vi "main_FP.vi"() -> ()   [LabVIEW 2011]
uses:
  global.vi
  <vilib>/Instr/_visa.llb/VISA Configure Serial Port (Instr).vi
panel:
  in  "EXIT":bool caption="Start_reception"
  out "status_error":bool caption="status_rx"
  out "status_tx":bool
  out "status_rx":bool
  out "status_connected":bool
  in  "Main tab":T1(tab)
  in  "Stop_rx":bool
  out "Receiving":bool
  out "Signal Noise Ratio":string="0"
  out "Packet number":i32
  in  "Start_reception":bool
  in  "reception_list":i32(listbox)
  out "reception Graph":dbl[](graph)
  in  "Stop_tx":bool
  out "Transmitting":bool
  in  "Delay between packets (ms)":u32=2000 max=65535 step=1
  in  "tx_timestamp":bool=TRUE caption="Add timestamp"
  in  "tx_packetnum":bool=TRUE caption="Add packet number"
  in  "Message":string="Aloha"
  out "TX Packet number":i32 caption="Packet number"
  in  "Start_transmission":bool
  in  "transmission_list":i32(listbox)
  in  "Bandwidth":string(combo)="125"
  in  "CRC":bool=TRUE
  in  "Preamble length":u32=8 max=65535 step=1
  in  "Frequency":u32=868100000 max=65535 step=1
  in  "Bitrate":u32=50000 max=65535 step=1
  in  "Freq deviation":u32=25000 max=65535 step=1
  in  "RX signal bw":string(combo)="25kHz"
  in  "Freq correct":string(combo)="41.7kHz"
  in  "Spreading factor":string(combo)="sf12"
  in  "Power":string(combo)="1"
  in  "Radio mode":string(combo)="lora"
  out "EUI address":string="\r\n"
  out "Voltage":string="\r\n"
  out "Version":string="\r\n"
  in  "Save_changes":bool
  in  "Cancel_changes":bool
  in  "Discover device":bool=TRUE
  in  "Timeout (ms)":u32=10000
  in  "Port":refnum<visa-resource-name>="COM1"
  in  "Parity":u16(ring) items=["None", "Odd", "Even", "Mark", "Space"]
  in  "Stop bits":u16(ring)=10 items=["1.0"=10, "1.5"=15, "2.0"=20]
  in  "Baud rate":u32=57600
  in  "Data bits":u16=8
  # "RN2483 LoRa transceiver utility"
  # "V0.9"
  # "Status"
  # "Reception mode"
  # "Transmission mode"
  # "Device info"
  # "Device config"
  # "Serial port"
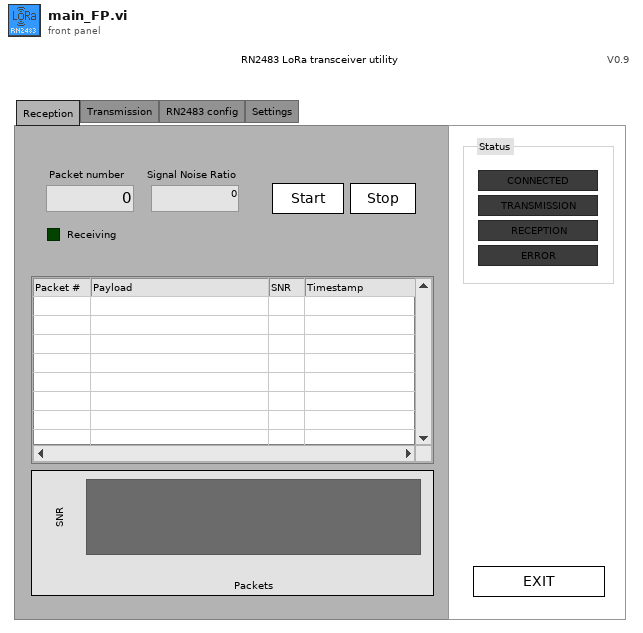
[diagram p1: front panel]
types:
  T1 = enum32{"Reception", "Transmission", "RN2483 config", "Settings"}
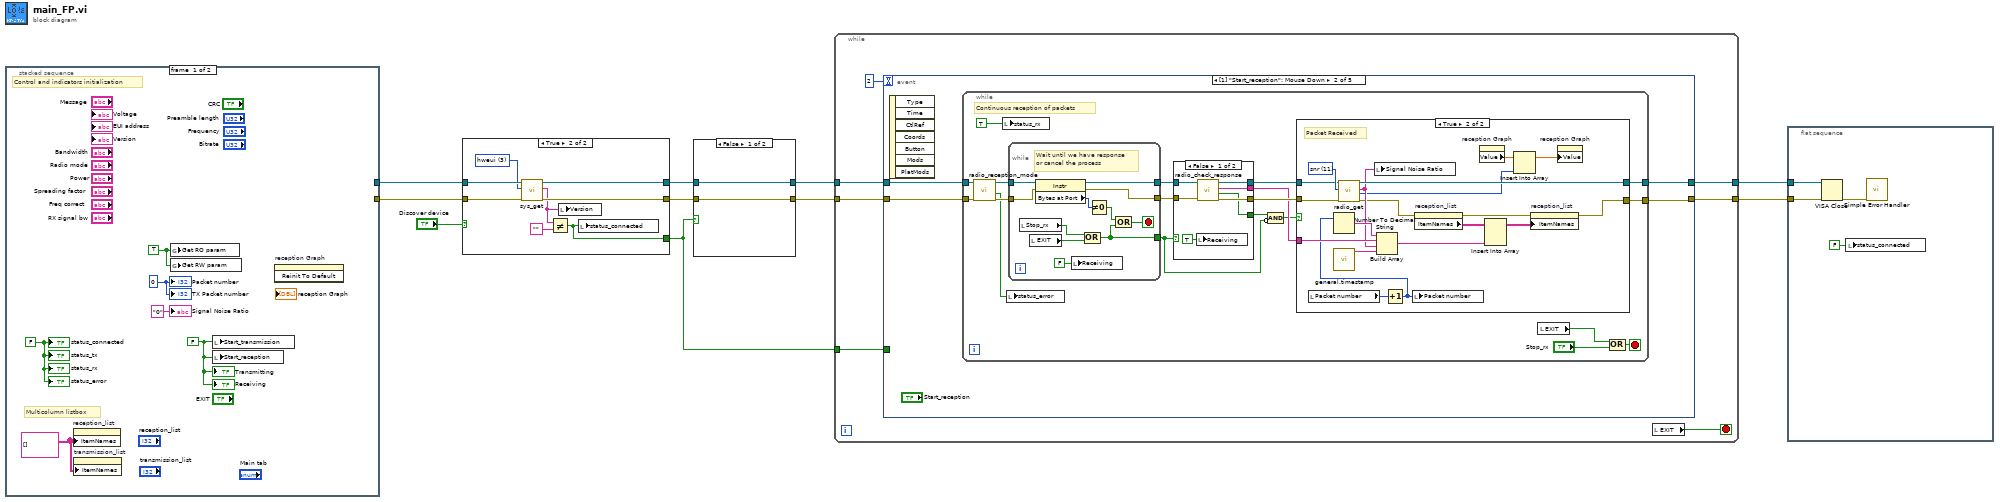
[diagram p0: block diagram]
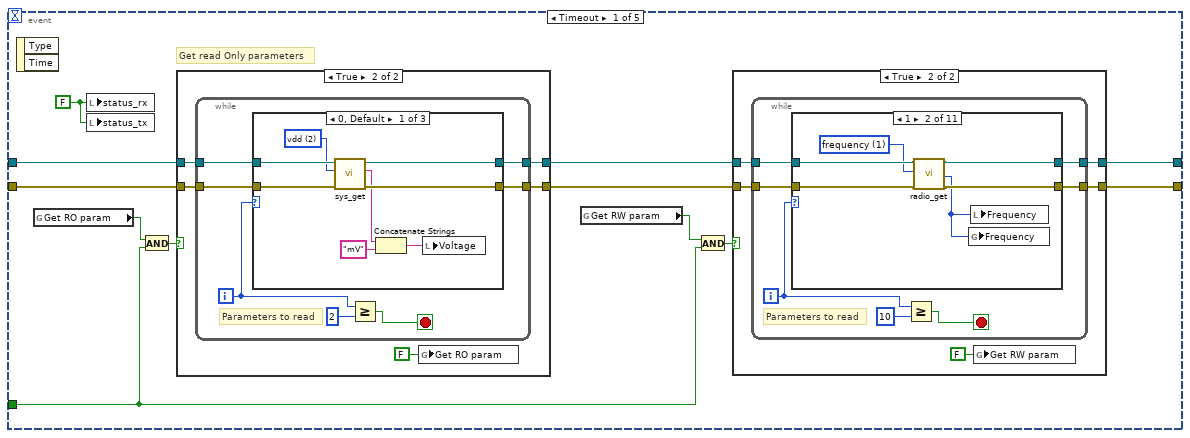
[diagram p2: hidden frame]
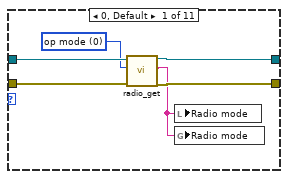
[diagram p4: hidden frame]
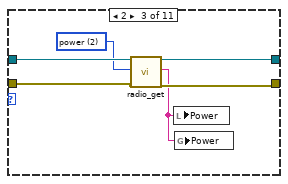
[diagram p5: hidden frame]
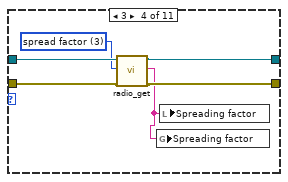
[diagram p6: hidden frame]
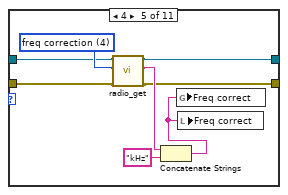
[diagram p7: hidden frame]
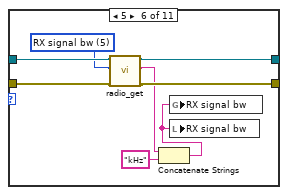
[diagram p8: hidden frame]
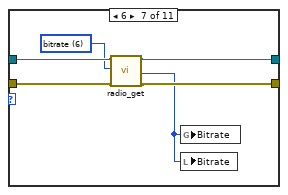
[diagram p9: hidden frame]
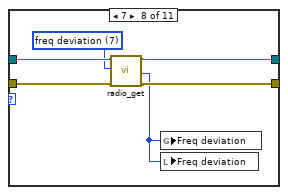
[diagram p10: hidden frame]
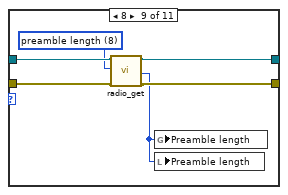
[diagram p11: hidden frame]
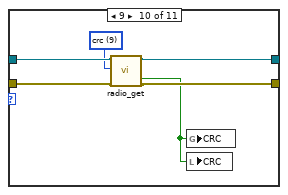
[diagram p12: hidden frame]
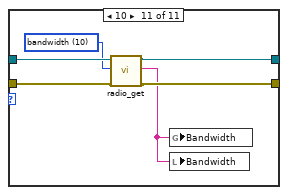
[diagram p13: hidden frame]
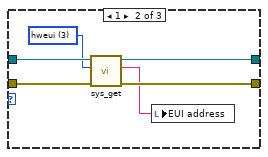
[diagram p15: hidden frame]
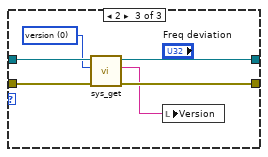
[diagram p16: hidden frame]
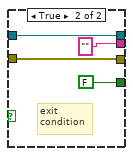
[diagram p17: hidden frame]
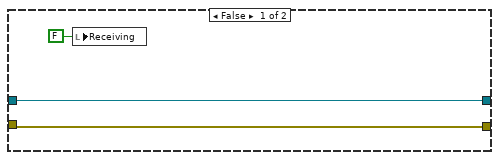
[diagram p18: hidden frame]
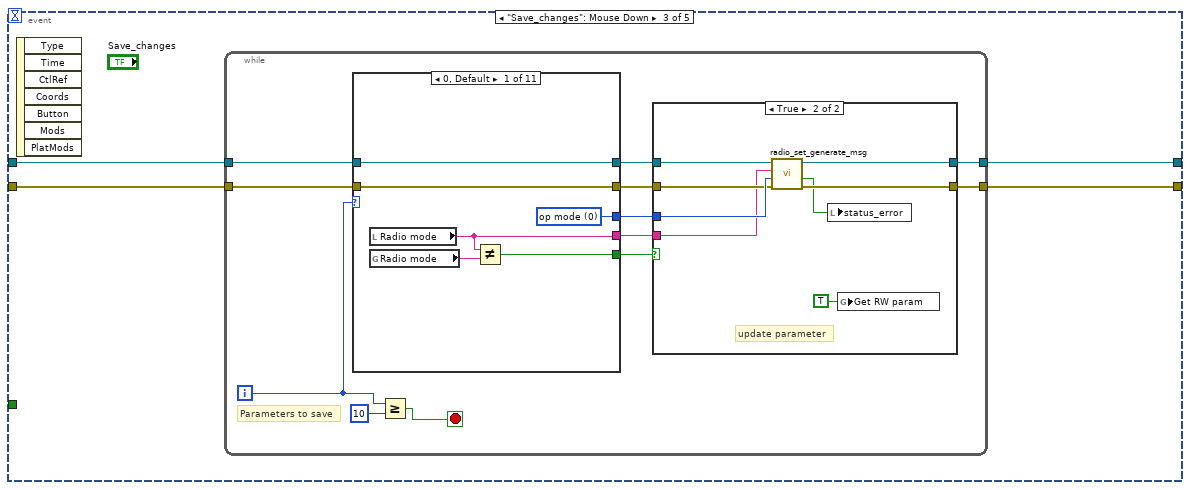
[diagram p19: hidden frame]
diagram:
  n1 = stacked-sequence {
    tunnel: [_ w19] -> w9
    tunnel: [_ w18] -> w8
    frame #0 {
      w12 = FALSE ("status_connected")
      w13 = string[][] [] ("Item Names")
      w11 = FALSE ("Receiving")
      w14 = 0 ("Packet number")
      w16 = TRUE ("Get RO param")
      # "Multicolumn listbox"
      # "Control and indicators initialization"
      n2 = property on="reception_list" class="MCListbox (strict)"("ItemNames"=w13) -> ()  [unwired: 2 in, 2 out]
      n3 = property on="transmission_list" class="MCListbox (strict)"("ItemNames"=w13) -> ()  [unwired: 2 in, 2 out]
      n4 = global write "global.vi" "Get RO param"(w16) -> ()
      n5 = global write "global.vi" "Get RW param"(w16) -> ()
      n6 = local write "Start_transmission"(w11) -> ()
      n7 = local write "Start_reception"(w11) -> ()
      n8 = invoke on="reception Graph" class="WFGraph (strict)" method="Reinit To Default"() -> ()  [unwired: 3 in, 3 out]
      "Packet number" <- w14
      "Signal Noise Ratio" <- "0" ("Signal Noise Ratio")
      "TX Packet number" <- w14
      "Transmitting" <- w11
      "status_connected" <- w12
      "status_tx" <- w12
      "status_rx" <- w12
      "status_error" <- w12
      "Receiving" <- w11
    }
    frame #1 {
      w22 = u16 0 items=["None", "XON/XOFF", "RTS/CTS", "DTR/DSR"] ("Flow control")
      # "Configure Serial port (baud rate, data bits, parity, stop bits and flow control)."
      n9 = call-poly "VISA Configure Serial Port"("VISA resource name"="Port", "timeout (10sec)"="Timeout (ms)", "baud rate (9600)"="Baud rate", "data bits (8)"="Data bits", "parity (0:none)"="Parity", "stop bits (10: 1 bit)"="Stop bits", "flow control (0:none)"=w22) -> ("VISA resource name out"=w19:refnum<visa-resource-name>, "error out"=w18:errorcluster)  [unwired: 2 in, 5 out]
    }
  }
  n10 = case shown="True" "Discover device" {
    tunnel: [w28 w34] -> w3
    tunnel: w9 -> [w27 w36]
    tunnel: w8 -> [w28 w35]
    tunnel: [w27 w33] -> w4
    tunnel: [FALSE w30] -> w5
    frame False {
    }
    frame True {
      w32 = u16 3 items=["version", "nvm", "vdd", "hweui"] ("Sys get command")
      n11 = call "sys_get.vi"("error in"=w35, "Sys get command"=w32, "VISA in"=w36) -> ("error out"=w34:errorcluster, "response"=w29:string, "VISA out"=w33:refnum<visa-resource-name>)  [unwired: 6 in]
      n12 = Not Equal?(x=w29, y="") -> (x != y?=w30:bool)
      n13 = local write "Version"(w29) -> ()
      n14 = local write "status_connected"(w30) -> ()
    }
  }
  n15 = case shown="False" w5 {
    tunnel: w4 -> [w38 w42]
    tunnel: w3 -> [w37 w41]
    tunnel: [w38 w40] -> w2
    tunnel: [w37 w39] -> w1
    frame False {
    }
    frame True {
      n16 = call "mac_pause.vi"("error in"=w41, "VISA in"=w42) -> ("error out"=w39:errorcluster, "VISA out"=w40:refnum<visa-resource-name>)  [unwired: 7 in, 1 out]
    }
  }
  n17 = while {
    tunnel: [w49] -> w7
    tunnel: [w48] -> w6
    tunnel: w5 -> [w46]
    tunnel: w2 -> [w45]
    tunnel: w1 -> [w44]
    stop <- w43 stop-if-true
    n18 = event shown="[1] \"Start_reception\": Mouse Down" {
      selector: _ -> [_ _ _ _ _]
      dyn-events: _ -> [_ _ _ _ _]
      timeout: 2 -> [_ _ _ _ _]
      tunnel: [w54 w181 w248 w358 w360] -> w49
      tunnel: [w53 w180 w247 w357 w359] -> w48
      tunnel: w46 -> [w52 _ _ _ _]
      tunnel: w45 -> [w61 w183 w250 w358 w362]
      tunnel: w44 -> [w60 w182 w249 w357 w361]
      event Timeout {
        w50 = FALSE ("status_rx")
        # "Get read Only parameters"
        n19 = event-data() -> ()  [unwired: 1 in, 2 out]
        n20 = global read "global.vi" "Get RO param"() -> (w58:bool)
        n21 = local write "status_rx"(w50) -> ()
        n22 = local write "status_tx"(w50) -> ()
        n23 = And(x=w58, y=w52) -> (x .and. y?=w59:bool)
        n24 = case shown="True" w59 {
          tunnel: w61 -> [w147 w152]
          tunnel: w60 -> [w146 w151]
          tunnel: [w147 w150] -> w56
          tunnel: [w146 w149] -> w55
          frame False {
            # "Don't read RN2483 parameters"
          }
          frame True {
            n25 = while {
              tunnel: w152 -> [w159]
              tunnel: w151 -> [w158]
              tunnel: [w157] -> w150
              tunnel: [w156] -> w149
              i -> [w153]
              stop <- w154 stop-if-true
              # "Parameters to read"
              n26 = case shown="0, Default" w153 {
                tunnel: w159 -> [w167 w173 w179]
                tunnel: w158 -> [w166 w172 w178]
                tunnel: [w165 w171 w177] -> w157
                tunnel: [w164 w170 w176] -> w156
                frame 0, Default {
                  w163 = u16 2 items=["version", "nvm", "vdd", "hweui"] ("Sys get command")
                  n27 = call "sys_get.vi"("error in"=w166, "Sys get command"=w163, "VISA in"=w167) -> ("error out"=w164:errorcluster, "response"=w161:string, "VISA out"=w165:refnum<visa-resource-name>)  [unwired: 6 in]
                  n28 = Concatenate Strings(w161, "mV" ("string")) -> (w160:string)
                  n29 = local write "Voltage"(w160) -> ()
                }
                frame 1 {
                  w169 = u16 3 items=["version", "nvm", "vdd", "hweui"] ("Sys get command")
                  n30 = call "sys_get.vi"("error in"=w172, "Sys get command"=w169, "VISA in"=w173) -> ("error out"=w170:errorcluster, "response"=w168:string, "VISA out"=w171:refnum<visa-resource-name>)  [unwired: 6 in]
                  n31 = local write "EUI address"(w168) -> ()
                }
                frame 2 {
                  w175 = u16 0 items=["version", "nvm", "vdd", "hweui"] ("Sys get command")
                  n32 = call "sys_get.vi"("error in"=w178, "Sys get command"=w175, "VISA in"=w179) -> ("error out"=w176:errorcluster, "response"=w174:string, "VISA out"=w177:refnum<visa-resource-name>)  [unwired: 6 in]
                  n33 = local write "Version"(w174) -> ()
                }
              }
              n34 = Greater Or Equal?(x=w153, y=2) -> (x >= y?=w154:bool)
            }
            n35 = global write "global.vi" "Get RO param"(FALSE ("Get RO param")) -> ()
          }
        }
        n36 = global read "global.vi" "Get RW param"() -> (w51:bool)
        n37 = And(x=w51, y=w52) -> (x .and. y?=w57:bool)
        n38 = case shown="True" w57 {
          tunnel: w56 -> [w63 w68]
          tunnel: w55 -> [w62 w67]
          tunnel: [w63 w66] -> w54
          tunnel: [w62 w65] -> w53
          frame False {
            # "Don't read RN2483 parameters"
          }
          frame True {
            n39 = while {
              tunnel: w68 -> [w75]
              tunnel: w67 -> [w74]
              tunnel: [w73] -> w66
              tunnel: [w72] -> w65
              i -> [w69]
              stop <- w70 stop-if-true
              # "Parameters to read"
              n40 = case shown="1" w69 {
                tunnel: w75 -> [w81 w86 w93 w98 w101 w110 w120 w126 w132 w138 w144]
                tunnel: w74 -> [w79 w87 w92 w99 w103 w114 w121 w127 w133 w139 w145]
                tunnel: [w78 w84 w90 w97 w106 w112 w118 w124 w130 w136 w143] -> w73
                tunnel: [w77 w83 w89 w96 w104 w113 w117 w123 w129 w135 w142] -> w72
                frame 0, Default {
                  w80 = u16 0 items=["op mode", "frequency", "power", "spread factor"] ("Radio get command")
                  n41 = call "radio_get.vi"("VISA in"=w81, "Radio get command"=w80, "error in"=w79) -> ("VISA out"=w78:refnum<visa-resource-name>, "response"=w76:string, "error out"=w77:errorcluster)  [unwired: 12 in, 2 out]
                  n42 = local write "Radio mode"(w76) -> ()
                  n43 = global write "global.vi" "Radio mode"(w76) -> ()
                }
                frame 1 {
                  w85 = u16 1 items=["op mode", "frequency", "power", "spread factor"] ("Radio get command")
                  n44 = call "radio_get.vi"("VISA in"=w86, "Radio get command"=w85, "error in"=w87) -> ("VISA out"=w84:refnum<visa-resource-name>, "Num out"=w82:u32, "error out"=w83:errorcluster)  [unwired: 12 in, 2 out]
                  n45 = global write "global.vi" "Frequency"(w82) -> ()
                  n46 = local write "Frequency"(w82) -> ()
                }
                frame 2 {
                  w91 = u16 2 items=["op mode", "frequency", "power", "spread factor"] ("Radio get command")
                  n47 = call "radio_get.vi"("VISA in"=w93, "Radio get command"=w91, "error in"=w92) -> ("VISA out"=w90:refnum<visa-resource-name>, "response"=w88:string, "error out"=w89:errorcluster)  [unwired: 12 in, 2 out]
                  n48 = local write "Power"(w88) -> ()
                  n49 = global write "global.vi" "Power"(w88) -> ()
                }
                frame 3 {
                  w95 = u16 3 items=["op mode", "frequency", "power", "spread factor"] ("Radio get command")
                  n50 = call "radio_get.vi"("VISA in"=w98, "Radio get command"=w95, "error in"=w99) -> ("VISA out"=w97:refnum<visa-resource-name>, "response"=w94:string, "error out"=w96:errorcluster)  [unwired: 12 in, 2 out]
                  n51 = global write "global.vi" "Spreading factor"(w94) -> ()
                  n52 = local write "Spreading factor"(w94) -> ()
                }
                frame 4 {
                  w102 = u16 4 items=["op mode", "frequency", "power", "spread factor", "freq correction", "RX signal bw"] ("Radio get command")
                  n53 = call "radio_get.vi"("VISA in"=w101, "Radio get command"=w102, "error in"=w103) -> ("VISA out"=w106:refnum<visa-resource-name>, "response"=w105:string, "error out"=w104:errorcluster)  [unwired: 12 in, 2 out]
                  n54 = Concatenate Strings(w105, "kHz" ("string")) -> (w100:string)
                  n55 = global write "global.vi" "Freq correct"(w100) -> ()
                  n56 = local write "Freq correct"(w100) -> ()
                }
                frame 5 {
                  w109 = u16 5 items=["op mode", "frequency", "power", "spread factor", "freq correction", "RX signal bw"] ("Radio get command")
                  n57 = call "radio_get.vi"("VISA in"=w110, "Radio get command"=w109, "error in"=w114) -> ("VISA out"=w112:refnum<visa-resource-name>, "response"=w111:string, "error out"=w113:errorcluster)  [unwired: 12 in, 2 out]
                  n58 = Concatenate Strings(w111, "kHz" ("string")) -> (w108:string)
                  n59 = global write "global.vi" "RX signal bw"(w108) -> ()
                  n60 = local write "RX signal bw"(w108) -> ()
                }
                frame 6 {
                  w119 = u16 6 items=["op mode", "frequency", "power", "spread factor", "freq correction", "RX signal bw", "bitrate", "freq deviation", "preamble length", "crc"] ("Radio get command")
                  n61 = call "radio_get.vi"("VISA in"=w120, "Radio get command"=w119, "error in"=w121) -> ("VISA out"=w118:refnum<visa-resource-name>, "Num out"=w116:u32, "error out"=w117:errorcluster)  [unwired: 12 in, 2 out]
                  n62 = global write "global.vi" "Bitrate"(w116) -> ()
                  n63 = local write "Bitrate"(w116) -> ()
                }
                frame 7 {
                  w125 = u16 7 items=["op mode", "frequency", "power", "spread factor", "freq correction", "RX signal bw", "bitrate", "freq deviation", "preamble length", "crc"] ("Radio get command")
                  n64 = call "radio_get.vi"("VISA in"=w126, "Radio get command"=w125, "error in"=w127) -> ("VISA out"=w124:refnum<visa-resource-name>, "Num out"=w122:u32, "error out"=w123:errorcluster)  [unwired: 12 in, 2 out]
                  n65 = global write "global.vi" "Freq deviation"(w122) -> ()
                  n66 = local write "Freq deviation"(w122) -> ()
                }
                frame 8 {
                  w131 = u16 8 items=["op mode", "frequency", "power", "spread factor", "freq correction", "RX signal bw", "bitrate", "freq deviation", "preamble length", "crc"] ("Radio get command")
                  n67 = call "radio_get.vi"("VISA in"=w132, "Radio get command"=w131, "error in"=w133) -> ("VISA out"=w130:refnum<visa-resource-name>, "Num out"=w128:u32, "error out"=w129:errorcluster)  [unwired: 12 in, 2 out]
                  n68 = global write "global.vi" "Preamble length"(w128) -> ()
                  n69 = local write "Preamble length"(w128) -> ()
                }
                frame 9 {
                  w137 = u16 9 items=["op mode", "frequency", "power", "spread factor", "freq correction", "RX signal bw", "bitrate", "freq deviation", "preamble length", "crc"] ("Radio get command")
                  n70 = call "radio_get.vi"("VISA in"=w138, "Radio get command"=w137, "error in"=w139) -> ("VISA out"=w136:refnum<visa-resource-name>, "Bool out"=w134:bool, "error out"=w135:errorcluster)  [unwired: 12 in, 2 out]
                  n71 = global write "global.vi" "CRC"(w134) -> ()
                  n72 = local write "CRC"(w134) -> ()
                }
                frame 10 {
                  w141 = u16 10 items=["op mode", "frequency", "power", "spread factor", "freq correction", "RX signal bw", "bitrate", "freq deviation", "preamble length", "crc", "bandwidth"] ("Radio get command")
                  n73 = call "radio_get.vi"("VISA in"=w144, "Radio get command"=w141, "error in"=w145) -> ("VISA out"=w143:refnum<visa-resource-name>, "response"=w140:string, "error out"=w142:errorcluster)  [unwired: 12 in, 2 out]
                  n74 = global write "global.vi" "Bandwidth"(w140) -> ()
                  n75 = local write "Bandwidth"(w140) -> ()
                }
              }
              n76 = Greater Or Equal?(x=w69, y=10) -> (x >= y?=w70:bool)
            }
            n77 = global write "global.vi" "Get RW param"(FALSE ("Get RO param")) -> ()
          }
        }
      }
      event "Start_reception": Mouse Down {
        n78 = event-data() -> ()  [unwired: 1 in, 7 out]
        n79 = while {
          tunnel: w183 -> [w201]
          tunnel: w182 -> [w202]
          tunnel: [w192] -> w181
          tunnel: [w191] -> w180
          stop <- w200 stop-if-true
          # "Continuous reception of packets"
          n80 = call "radio_reception_mode.vi"("error in"=w202, "VISA in"=w201) -> ("error out"=w198:errorcluster, "error"=w189:bool, "VISA out"=w199:refnum<visa-resource-name>)  [unwired: 7 in]
          n81 = local write "status_rx"(TRUE ("Receiving")) -> ()
          n82 = local write "status_error"(w189) -> ()
          n83 = while {
            tunnel: w199 -> [w246]
            tunnel: w198 -> [w245]
            tunnel: [w244] -> w196
            tunnel: [w243] -> w197
            tunnel: [w238] -> w185
            stop <- w240 stop-if-true
            # "Wait until we have response\nor cancel the process"
            n84 = local read "Stop_rx"() -> (w239:bool)
            n85 = local read "EXIT"() -> (w237:bool)
            n86 = property class="Instr"(reference=w246, error in=w245) -> (reference out=w244:refnum<visa-resource-name>, error out=w243:errorcluster, "Bytes at Port"=w242:u32)
            n87 = local write "Receiving"(FALSE ("Receiving")) -> ()
            n88 = Compound Arithmetic op=OR(w239, w237) -> (w238:bool)
            n89 = Not Equal To 0?(x=w242) -> (x != 0?=w241:bool)
            n90 = Compound Arithmetic op=OR(w241, w238) -> (w240:bool)
          }
          n91 = case shown="False" w185 {
            tunnel: w197 -> [w209 w212]
            tunnel: w196 -> [w208 w213]
            tunnel: [w207 w212] -> w195
            tunnel: [w206 w213] -> w194
            tunnel: [w205 "" ("read buffer")] -> w193
            tunnel: [w204 FALSE ("ok")] -> w184
            frame False {
              n92 = local write "Receiving"(TRUE ("Receiving")) -> ()
              n93 = call "radio_check_response.vi"("error in"=w209, "VISA in"=w208) -> ("error out"=w207:errorcluster, "ok"=w204:bool, "read buffer"=w205:string, "VISA out"=w206:refnum<visa-resource-name>)  [unwired: 6 in]
            }
            frame True {
              # "exit\ncondition"
            }
          }
          n94 = Compound Arithmetic op=AND(w184, invert w185) -> (w186:bool)
          n95 = case shown="True" w186 {
            tunnel: w195 -> [w215 w229]
            tunnel: w194 -> [w216 w230]
            tunnel: w193 -> [_ w232]
            tunnel: [w215 w217] -> w191
            tunnel: [w216 w228] -> w192
            frame False {
              n96 = local write "Receiving"(FALSE ("Receiving")) -> ()
            }
            frame True {
              w231 = u16 11 items=["op mode", "frequency", "power", "spread factor", "freq correction", "RX signal bw", "bitrate", "freq deviation", "preamble length", "crc", "bandwidth", "snr"] ("Radio get command")
              # "Packet Received"
              n97 = local read "Packet number"() -> (w235:i32)
              n98 = call "general.timestamp.vi"() -> ("timestamp"=w227:string)  [unwired: 11 in]
              n99 = call "radio_get.vi"("VISA in"=w230, "Radio get command"=w231, "error in"=w229) -> ("VISA out"=w228:refnum<visa-resource-name>, "response"=w223:string, "Num out"=w221:u32, "error out"=w219:errorcluster)  [unwired: 12 in, 1 out]
              n100 = local write "Signal Noise Ratio"(w223) -> ()
              n101 = Increment(x=w235) -> (x+1=w224:i32)
              n102 = Number To Decimal String(number=w224) -> (decimal integer string=w233:string)  [unwired: 1 in]
              n103 = Build Array(w233, w232, w223, w227) -> (w226:string[])
              n104 = local write "Packet number"(w224) -> ()
              n105 = property on="reception_list" class="MCListbox (strict)"(error in=w219) -> (error out=w218:errorcluster, "ItemNames"=w234:string[][])  [unwired: 1 in, 1 out]
              n106 = property on="reception Graph" class="WFGraph (strict)"() -> ("Value"=w222:dbl[])  [unwired: 2 in, 2 out]
              n107 = Insert Into Array(array=w234, new element=w226) -> (w225:string[][])  [unwired: 2 in]
              n108 = Insert Into Array(array=w222, new element=w221) -> (w220:dbl[])  [unwired: 1 in]
              n109 = property on="reception_list" class="MCListbox (strict)"(error in=w218, "ItemNames"=w225) -> (error out=w217:errorcluster)  [unwired: 1 in, 1 out]
              n110 = property on="reception Graph" class="WFGraph (strict)"("Value"=w220) -> ()  [unwired: 2 in, 2 out]
            }
          }
          n111 = local read "EXIT"() -> (w188:bool)
          n112 = Compound Arithmetic op=OR(w188, "Stop_rx") -> (w200:bool)
        }
      }
      event "Save_changes": Mouse Down {
        n113 = event-data() -> ()  [unwired: 1 in, 7 out]
        n114 = while {
          tunnel: w250 -> [w262]
          tunnel: w249 -> [w261]
          tunnel: [w255] -> w248
          tunnel: [w254] -> w247
          i -> [w258]
          stop <- w259 stop-if-true
          # "Parameters to save"
          n115 = case shown="0, Default" w258 {
            tunnel: w262 -> [w275 w280 w287 w293 w299 w305 w311 w318 w325 w337 w341]
            tunnel: w261 -> [w274 w279 w286 w292 w298 w304 w310 w317 w324 w336 w340]
            tunnel: [w275 w280 w287 w293 w299 w305 w311 w318 w325 w337 w341] -> w257
            tunnel: [w274 w279 w286 w292 w298 w304 w310 w317 w324 w336 w340] -> w256
            tunnel: [w277 w284 w290 w296 w302 w308 w315 w322 w329 w335 w344] -> w253
            tunnel: [w273 w281 w288 w294 w300 w306 w312 w319 w326 w331 w342] -> w252
            tunnel: [w276 w283 w289 w295 w301 w307 w314 w321 w328 w338 w343] -> w251
            frame 0, Default {
              w276 = u16 0 items=["op mode", "frequency", "power", "spread factor", "freq correction", "RX signal bw", "bitrate", "freq deviation", "preamble length", "crc", "bandwidth"] ("Radio get command")
              n116 = local read "Radio mode"() -> (w273:string)
              n117 = global read "global.vi" "Radio mode"() -> (w278:string)
              n118 = Not Equal?(x=w273, y=w278) -> (x != y?=w277:bool)
            }
            frame 1 {
              w283 = u16 1 items=["op mode", "frequency", "power", "spread factor", "freq correction", "RX signal bw", "bitrate", "freq deviation", "preamble length", "crc", "bandwidth"] ("Radio get command")
              n119 = global read "global.vi" "Frequency"() -> (w285:u32)
              n120 = local read "Frequency"() -> (w282:u32)
              n121 = Not Equal?(x=w282, y=w285) -> (x != y?=w284:bool)
              n122 = Number To Decimal String(number=w282) -> (decimal integer string=w281:string)  [unwired: 1 in]
            }
            frame 2 {
              w289 = u16 2 items=["op mode", "frequency", "power", "spread factor", "freq correction", "RX signal bw", "bitrate", "freq deviation", "preamble length", "crc", "bandwidth"] ("Radio get command")
              n123 = local read "Power"() -> (w288:string)
              n124 = global read "global.vi" "Power"() -> (w291:string)
              n125 = Not Equal?(x=w288, y=w291) -> (x != y?=w290:bool)
            }
            frame 3 {
              w295 = u16 3 items=["op mode", "frequency", "power", "spread factor", "freq correction", "RX signal bw", "bitrate", "freq deviation", "preamble length", "crc", "bandwidth"] ("Radio get command")
              n126 = local read "Spreading factor"() -> (w294:string)
              n127 = global read "global.vi" "Spreading factor"() -> (w297:string)
              n128 = Not Equal?(x=w294, y=w297) -> (x != y?=w296:bool)
            }
            frame 4 {
              w301 = u16 4 items=["op mode", "frequency", "power", "spread factor", "freq correction", "RX signal bw", "bitrate", "freq deviation", "preamble length", "crc", "bandwidth"] ("Radio get command")
              n129 = local read "Freq correct"() -> (w300:string)
              n130 = global read "global.vi" "Freq correct"() -> (w303:string)
              n131 = Not Equal?(x=w300, y=w303) -> (x != y?=w302:bool)
            }
            frame 5 {
              w307 = u16 5 items=["op mode", "frequency", "power", "spread factor", "freq correction", "RX signal bw", "bitrate", "freq deviation", "preamble length", "crc", "bandwidth"] ("Radio get command")
              n132 = local read "RX signal bw"() -> (w306:string)
              n133 = global read "global.vi" "RX signal bw"() -> (w309:string)
              n134 = Not Equal?(x=w306, y=w309) -> (x != y?=w308:bool)
            }
            frame 6 {
              w314 = u16 6 items=["op mode", "frequency", "power", "spread factor", "freq correction", "RX signal bw", "bitrate", "freq deviation", "preamble length", "crc", "bandwidth"] ("Radio get command")
              n135 = local read "Bitrate"() -> (w313:u32)
              n136 = global read "global.vi" "Bitrate"() -> (w316:u32)
              n137 = Not Equal?(x=w313, y=w316) -> (x != y?=w315:bool)
              n138 = Number To Decimal String(number=w313) -> (decimal integer string=w312:string)  [unwired: 1 in]
            }
            frame 7 {
              w321 = u16 7 items=["op mode", "frequency", "power", "spread factor", "freq correction", "RX signal bw", "bitrate", "freq deviation", "preamble length", "crc", "bandwidth"] ("Radio get command")
              n139 = global read "global.vi" "Freq deviation"() -> (w323:u32)
              n140 = local read "Freq deviation"() -> (w320:u32)
              n141 = Not Equal?(x=w320, y=w323) -> (x != y?=w322:bool)
              n142 = Number To Decimal String(number=w320) -> (decimal integer string=w319:string)  [unwired: 1 in]
            }
            frame 8 {
              w328 = u16 8 items=["op mode", "frequency", "power", "spread factor", "freq correction", "RX signal bw", "bitrate", "freq deviation", "preamble length", "crc", "bandwidth"] ("Radio get command")
              n143 = global read "global.vi" "Preamble length"() -> (w330:u32)
              n144 = local read "Preamble length"() -> (w327:u32)
              n145 = Not Equal?(x=w327, y=w330) -> (x != y?=w329:bool)
              n146 = Number To Decimal String(number=w327) -> (decimal integer string=w326:string)  [unwired: 1 in]
            }
            frame 9 {
              w338 = u16 8 items=["op mode", "frequency", "power", "spread factor", "freq correction", "RX signal bw", "bitrate", "freq deviation", "preamble length", "crc", "bandwidth"] ("Radio get command")
              n147 = global read "global.vi" "CRC"() -> (w339:bool)
              n148 = local read "CRC"() -> (w334:bool)
              n149 = Not Equal?(x=w334, y=w339) -> (x != y?=w335:bool)
              n150 = Select(t="on", s=w334, f="off") -> (s? t:f=w331:string)
            }
            frame 10 {
              w343 = u16 10 items=["op mode", "frequency", "power", "spread factor", "freq correction", "RX signal bw", "bitrate", "freq deviation", "preamble length", "crc", "bandwidth"] ("Radio get command")
              n151 = local read "Bandwidth"() -> (w342:string)
              n152 = global read "global.vi" "Bandwidth"() -> (w345:string)
              n153 = Not Equal?(x=w342, y=w345) -> (x != y?=w344:bool)
            }
          }
          n154 = Greater Or Equal?(x=w258, y=10) -> (x >= y?=w259:bool)
          n155 = case shown="True" w253 {
            tunnel: [w264 w269] -> w255
            tunnel: [w263 w268] -> w254
            tunnel: w257 -> [w264 w271]
            tunnel: w256 -> [w263 w270]
            tunnel: w252 -> [_ w267]
            tunnel: w251 -> [_ w272]
            frame False {
              # "Parameter not changed,\ndo nothing"
            }
            frame True {
              # "update parameter"
              n156 = call "radio_set_generate_msg.vi"("error in"=w270, "Radio command"=w272, "input parameter"=w267, "VISA in"=w271) -> ("error out"=w268:errorcluster, "error"=w265:bool, "VISA out"=w269:refnum<visa-resource-name>)  [unwired: 4 in, 1 out]
              n157 = local write "status_error"(w265) -> ()
              n158 = global write "global.vi" "Get RW param"(TRUE ("Get RW param")) -> ()
            }
          }
        }
      }
      event "Cancel_changes": Mouse Down {
        n159 = event-data() -> ()  [unwired: 1 in, 7 out]
        n160 = global read "global.vi" "Spreading factor"() -> (w354:string)
        n161 = global read "global.vi" "Preamble length"() -> (w349:u32)
        n162 = global read "global.vi" "Freq deviation"() -> (w350:u32)
        n163 = global read "global.vi" "RX signal bw"() -> (w352:string)
        n164 = global read "global.vi" "Radio mode"() -> (w346:string)
        n165 = global read "global.vi" "Freq correct"() -> (w353:string)
        n166 = global read "global.vi" "Bandwidth"() -> (w347:string)
        n167 = global read "global.vi" "Frequency"() -> (w356:u32)
        n168 = global read "global.vi" "Bitrate"() -> (w351:u32)
        n169 = global read "global.vi" "Power"() -> (w355:string)
        n170 = global read "global.vi" "CRC"() -> (w348:bool)
        n171 = local write "Frequency"(w356) -> ()
        n172 = local write "Power"(w355) -> ()
        n173 = local write "Spreading factor"(w354) -> ()
        n174 = local write "Freq correct"(w353) -> ()
        n175 = local write "RX signal bw"(w352) -> ()
        n176 = local write "Bitrate"(w351) -> ()
        n177 = local write "Freq deviation"(w350) -> ()
        n178 = local write "Preamble length"(w349) -> ()
        n179 = local write "CRC"(w348) -> ()
        n180 = local write "Bandwidth"(w347) -> ()
        n181 = local write "Radio mode"(w346) -> ()
      }
      event "Start_transmission": Mouse Down {
        n182 = event-data() -> ()  [unwired: 1 in, 5 out]
        n183 = while {
          tunnel: w362 -> [w392]
          tunnel: w361 -> [w391]
          tunnel: [w394] -> w360
          tunnel: [w393] -> w359
          i -> [w368]
          stop <- w395 stop-if-true
          w366 = TRUE ("Receiving")
          # "Continuous transmission of packets"
          n184 = local read "Message"() -> (w388:string)
          n185 = call "general.timestamp.vi"() -> ("timestamp"=w380:string)  [unwired: 11 in]
          n186 = local write "Transmitting"(w366) -> ()
          n187 = Number To Decimal String(number=w368) -> (decimal integer string=w382:string)  [unwired: 1 in]
          n188 = local write "status_tx"(w366) -> ()
          n189 = Concatenate Strings(w382, "_" ("element")) -> (w383:string)
          n190 = Concatenate Strings(w388, "_" ("element")) -> (w386:string)
          n191 = Empty String/Path?(string/path=w388) -> (empty?=w390:bool)
          n192 = Concatenate Strings(w380, "_" ("element")) -> (w377:string)
          n193 = Select(t=w383, s="tx_packetnum", f="") -> (s? t:f=w375:string)
          n194 = Select(t="", s=w390, f=w386) -> (s? t:f=w374:string)
          n195 = Select(t=w377, s="tx_timestamp", f="") -> (s? t:f=w373:string)
          n196 = Concatenate Strings(w374, w375, w373) -> (w370:string)
          n197 = call "general.ascii2hex.vi"("Ascii input Message"=w370) -> ("Hex output Message"=w369:string)  [unwired: 10 in]
          n198 = call "radio_transmission_mode.vi"("error in"=w391, "message"=w369, "VISA in"=w392) -> ("error out"=w371:errorcluster, "error"=w365:bool, "VISA out"=w372:refnum<visa-resource-name>)  [unwired: 6 in]
          n199 = local write "TX Packet number"(w368) -> ()
          n200 = local write "status_error"(w365) -> ()
          n201 = case shown="False" w365 {
            tunnel: w371 -> [w397 w409]
            tunnel: w372 -> [w403 w410]
            tunnel: w370 -> [w406 _]
            tunnel: [w401 w409] -> w393
            tunnel: [w403 w410] -> w394
            tunnel: w368 -> [w404 _]
            frame False {
              # "Packet transmitted succesfully"
              n202 = local write "Transmitting"(FALSE ("Receiving")) -> ()
              n203 = Number To Decimal String(number=w404) -> (decimal integer string=w407:string)  [unwired: 1 in]
              n204 = call "general.timestamp.vi"() -> ("timestamp"=w402:string)  [unwired: 11 in]
              n205 = Build Array(w407, w406, w402) -> (w405:string[])
              n206 = property on="transmission_list" class="MCListbox (strict)"(error in=w397) -> (error out=w398:errorcluster, "ItemNames"=w400:string[][])  [unwired: 1 in, 1 out]
              n207 = Insert Into Array(array=w400, new element=w405) -> (w399:string[][])  [unwired: 2 in]
              n208 = property on="transmission_list" class="MCListbox (strict)"(error in=w398, "ItemNames"=w399) -> (error out=w401:errorcluster)  [unwired: 1 in, 1 out]
            }
            frame True {
              n209 = local write "Transmitting"(FALSE ("Receiving")) -> ()
            }
          }
          n210 = local read "EXIT"() -> (w364:bool)
          n211 = Compound Arithmetic op=OR(w364, "Stop_tx") -> (w395:bool)
          n212 = Wait (ms)(milliseconds to wait="Delay between packets (ms)") -> ()  [unwired: 1 out]
        }
      }
    }
    n213 = local read "EXIT"() -> (w43:bool)
  }
  n214 = flat-sequence {
    tunnel: w7 -> [w413]
    tunnel: w6 -> [w412]
    frame #0 {
      n215 = VISA Close(VISA resource name=w413, error in (no error)=w412) -> (error out=w414:errorcluster)
      n216 = local write "status_connected"(FALSE ("status_connected")) -> ()
      n217 = call <vilib>:"Simple Error Handler.vi"("error in (no error)"=w414) -> ()  [unwired: 1 in, 8 out]
    }
  }
